vi "Digio Trigger Config.vi"(5 "Pulse Width (10e-6)":dbl=1e-05, 7 "Mode (Falling Edge)":T1(ring), 8 "error in":errorcluster, 9 "Line (1)":u32=1 min=1 max=14, 10 "Node In":string, 11 "VISA resource name":refnum<visa-resource-name>) -> (0 "error out":errorcluster, 2 "Node Out":string, 3 "VISA resource name out":refnum<visa-resource-name>, 4 "Command String":string)   [LabVIEW 2012, in "Keithley 2600 Series.lvlib"]
doc: "This VI configures a digital I/O trigger line.\n\n<b>Functions and Attributes Used</b>\ndigio.trigger[n].mode\ndigio.trigger[n].pulsewidth\n\nNote:\nDigital IO feature is not supported with Keithley 2604B, 2614B, 2634B."
uses:
  Keithley 2600 Series.lvlib
  Private/GlobalVariables.vi
panel:
  # "(c) 2008 Keithley Instruments, Inc.  ALL RIGHTS RESERVED."
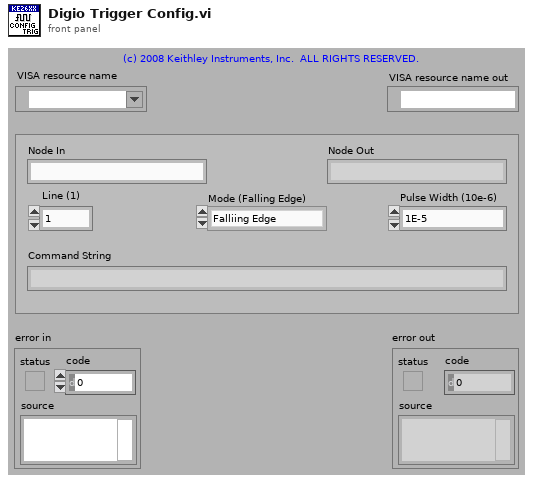
[diagram p1: front panel]
types:
  T1 = enum16{"Falliing Edge", "Rising Edge", "Rising or Falling", "Synchronous"}
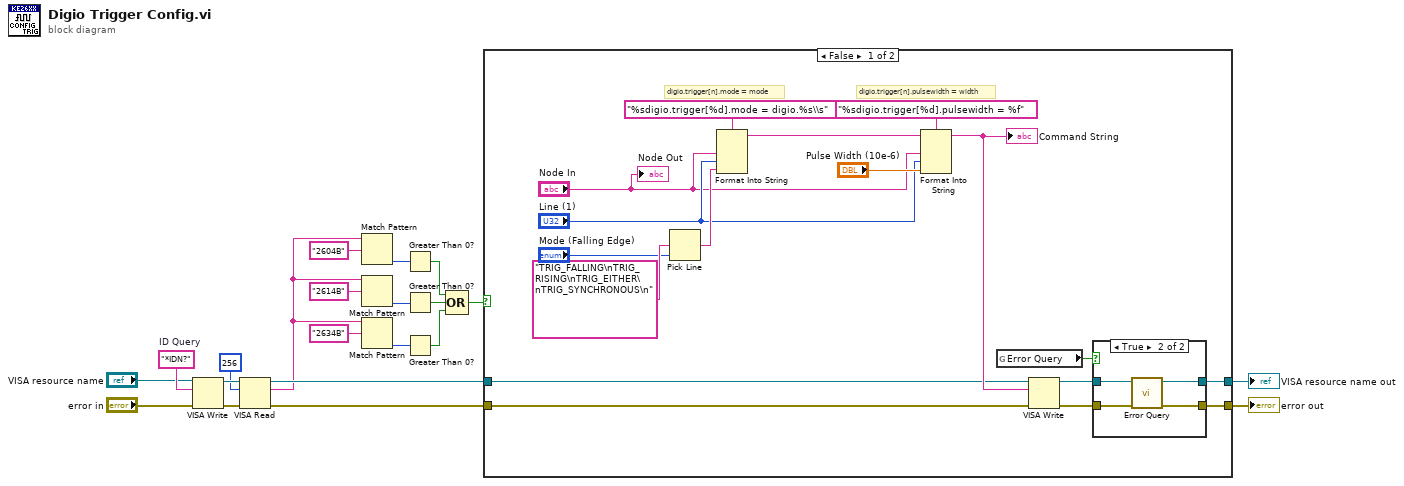
[diagram p0: block diagram]
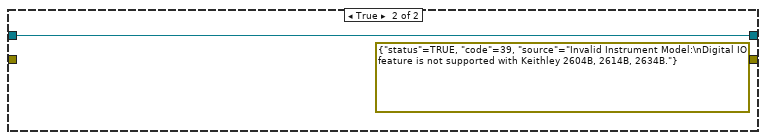
[diagram p3: hidden frame]
diagram:
  w15 = "*IDN?"  # ID Query
  n1 = VISA Write(VISA resource name="VISA resource name", write buffer=w15, error in (no error)="error in") -> (VISA resource name out=w19:refnum<visa-resource-name>, error out=w18:errorcluster)  [unwired: 1 out]
  n2 = VISA Read(VISA resource name=w19, byte count=u32 256, error in (no error)=w18) -> (VISA resource name out=w16:refnum<visa-resource-name>, read buffer=w1:string, error out=w14:errorcluster)  [unwired: 1 out]
  n3 = Match Pattern(string=w1, regular expression="2604B" ("y")) -> (offset past match=w8:i32)  [unwired: 1 in, 3 out]
  n4 = Match Pattern(string=w1, regular expression="2614B" ("y")) -> (offset past match=w7:i32)  [unwired: 1 in, 3 out]
  n5 = Match Pattern(string=w1, regular expression="2634B" ("y")) -> (offset past match=w6:i32)  [unwired: 1 in, 3 out]
  n6 = Greater Than 0?(x=w8) -> (x > 0?=w5:bool)
  n7 = Greater Than 0?(x=w7) -> (x > 0?=w4:bool)
  n8 = Greater Than 0?(x=w6) -> (x > 0?=w3:bool)
  n9 = Compound Arithmetic op=OR(w5, w4, w3) -> (w2:bool)
  n10 = case shown="False" w2 {
    tunnel: [w26 w46] -> w21
    tunnel: [w25 errorcluster {"status"=TRUE, "code"=39, "source"="Invalid Instrument Model:\nDigital IO feature is not supported with Keithley 2604B, 2614B, 2634B."} ("error out")] -> w20
    tunnel: w16 -> [w23 w46]
    tunnel: w14 -> [w22 _]
    frame False {
      # "digio.trigger[n].pulsewidth = width"
      # "digio.trigger[n].mode = mode"
      n11 = Pick Line(multi-line string="TRIG_FALLING\nTRIG_RISING\nTRIG_EITHER\nTRIG_SYNCHRONOUS\n", line index="Mode (Falling Edge)") -> (output string=w35:string)  [unwired: 1 out]
      n12 = Format Into String(format string="%sdigio.trigger[%d].mode = digio.%s\\s", "Node In", "Line (1)", w35) -> (resulting string=w31:string)  [unwired: 2 in, 1 out]
      n13 = Format Into String(format string="%sdigio.trigger[%d].pulsewidth = %f", initial string=w31, "Node In", "Line (1)", "Pulse Width (10e-6)") -> (resulting string=w24:string)  [unwired: 1 in, 1 out]
      "Command String" <- w24
      n14 = global read "GlobalVariables.vi" "Error Query"() -> (w27:bool)
      n15 = VISA Write(VISA resource name=w23, write buffer=w24, error in (no error)=w22) -> (VISA resource name out=w29:refnum<visa-resource-name>, error out=w28:errorcluster)  [unwired: 1 out]
      n16 = case shown="True" w27 {
        tunnel: w29 -> [w40 w44]
        tunnel: w28 -> [w39 w43]
        tunnel: [w40 w42] -> w26
        tunnel: [w39 w41] -> w25
        frame False {
        }
        frame True {
          n17 = call "Error Query.vi"("error in (no error)"=w43, "VISA resource name"=w44) -> ("error out"=w41:errorcluster, "VISA resource name out"=w42:refnum<visa-resource-name>)  [unwired: 8 out]
        }
      }
      "Node Out" <- "Node In"
    }
    frame True {
    }
  }
  "VISA resource name out" <- w21
  "error out" <- w20
